vi "createCameraOutputMatrix.vi"(2 "Camera.lvclass":refnum<class "Camera.lvclass">, 3 "Scan.lvclass":refnum<class "Scan.lvclass">) -> (1 "raw":u16[][][][](array[numeric]))   [LabVIEW 2017]
uses:
  classes/Scans/Scan.lvclass
  classes/HardwareObjects/Camera/Camera.lvclass
  classes/Scans/Scan.lvclass/Scan.ctl
  classes/HardwareObjects/Camera/Camera.lvclass/Camera.ctl
  classes/Scans/Read A scans.vi
  classes/Scans/Read Bidirectional.vi
  classes/Scans/Read B scans.vi
  classes/Scans/Read Repeat B scans.vi
  classes/Scans/Read C scans.vi
  classes/HardwareObjects/Camera/Read Data Representation.vi
  classes/HardwareObjects/Camera/Read Camera Dimensions.vi
  classes/Scans/Read Scan Pattern.vi
panel:
  out "size(s)":i32[](array[numeric])
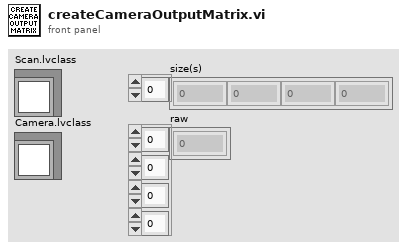
[diagram p1: front panel]
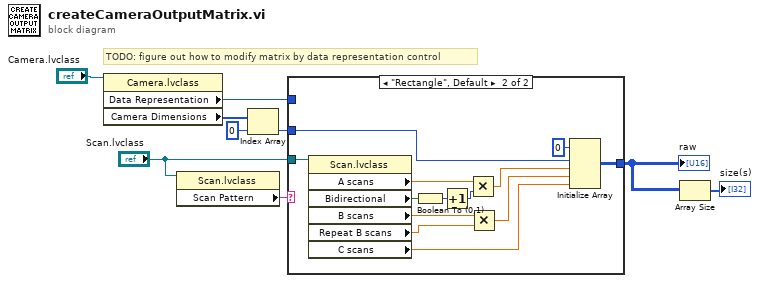
[diagram p0: block diagram]
diagram:
  # "TODO: figure out how to modify matrix by data representation control"
  n1 = property class="Camera.lvclass"(reference="Camera.lvclass") -> ("Data Representation"=w3:enum16{"U8", "I8", "U16", "I16"}, "Camera Dimensions"=w4:u16[])  [unwired: 1 in, 2 out]
  n2 = property class="Scan.lvclass"(reference="Scan.lvclass") -> ("Scan Pattern"=w9:string)  [unwired: 1 in, 2 out]
  n3 = Index Array(array=w4, index=0) -> (element=w5:u16)
  n4 = case shown="\"Rectangle\", Default" w9 {
    tunnel: "Scan.lvclass" -> [_ w22]
    tunnel: w5 -> [_ w12]
    tunnel: w3 -> [_ _]
    tunnel: [_ w10] -> w2
    frame "False" {
    }
    frame "Rectangle", Default {
      n5 = property class="Scan.lvclass"(reference=w22) -> ("A scans"=w18:dbl, "Bidirectional"=w21:bool, "B scans"=w17:dbl, "Repeat B scans"=w16:dbl, "C scans"=w14:dbl)  [unwired: 1 in, 2 out]
      n6 = Boolean To (0,1)(Boolean=w21) -> (0, 1=w20:i16)
      n7 = Increment(x=w20) -> (x+1=w19:i16)
      n8 = Multiply(x=w18, y=w19) -> (x*y=w13:dbl)
      n9 = Multiply(x=w17, y=w16) -> (x*y=w15:dbl)
      n10 = Initialize Array(u16 0, w12, w13, w15, w14) -> (w10:u16[][][][])
    }
  }
  "raw" <- w2
  n11 = Array Size(array=w2) -> (size(s)=→"size(s)":i32[])
